vi "Sigmoid function.vi"(1 "x":dbl format="%.2f") -> (0 "y=f(x) sigmoid":dbl format="%.2f")   [LabVIEW 2010]
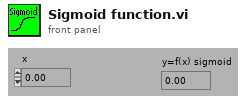
[diagram p1: front panel]
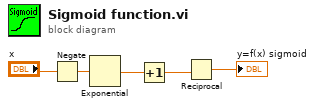
[diagram p0: block diagram]
diagram:
  n1 = Negate(x="x") -> (-x=w4:dbl)
  n2 = Exponential(1:w4) -> (0:w3:dbl)
  n3 = Increment(x=w3) -> (x+1=w2:dbl)
  n4 = Reciprocal(x=w2) -> (1/x=→"y=f(x) sigmoid":dbl)
